vi "_Construct Lens Values.vi"(7 "Lens List":i32[](array[numeric])) -> (2 "# of Lens":i32, 3 "Table":string[][](table))   [LabVIEW 2012]
uses:
  Type/_Run Module.ctl
  Configuration/_Global Configuration.vi
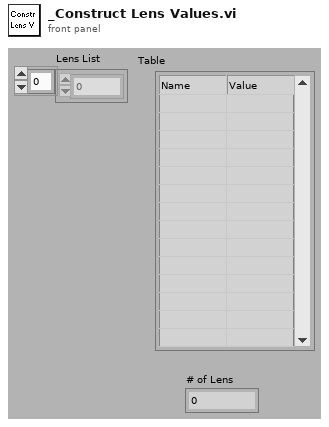
[diagram p1: front panel]
types:
  T1 = typedef "_Run Module.ctl" = u16
  T2 = typedef "_Lens Property.ctl" = cluster{"Scan Type":u8, "Scans":i32, "Time 1":dbl, "Time 2":dbl, "Value 1":dbl, "Value 2":dbl, "Step Size":dbl}
  T3 = typedef "_Mass Range Property.ctl" = cluster{"Start":dbl, "Stop":dbl, "Step Size":dbl, "Steps":i32, "Dwell":dbl, "Parameters":T4[], "Res":T5}
  T4 = typedef "_Mass Range Parameters.ctl" = cluster{"Name":string, "Ch#":u8, "StartV":dbl, "StopV":dbl, "StepV":dbl, "Index":u8}
  T5 = typedef "_RT Res Type.ctl" = u16
  T6 = typedef "_Run Mode.ctl" = enum16{"MRM (Q1/Q2)", "Q1 Scan", "Q1 SRM", "Q2 Scan", "Q2 SRM", "Product Scan", "Precursor Scan", "Neutral Loss", "Neutral Gain"}
  T7 = cluster{"Lenses":T2[], "Mass Ranges":T3[], "Acquire":bool, "MCA":bool, "Q1DC EN":bool, "Q1 POL":bool, "Q3 POL":bool, "Q1 RF  EN":bool, "Averaging":bool, "Log Scale":bool, "CPS":bool, "Unit":bool, "Data Path":path, "Run Mode":T6, "Fixed Mass (amu)":dbl, "Q3DC EN":bool, "Q3 RF  EN":bool, "Negative":bool}
  T8 = typedef "_RT Configuration 2.ctl" = cluster{"Name":string, "Ch#":u8, "Min":dbl, "Max":dbl, "Def+":dbl, "Def-":dbl, "Offset":dbl, "Slope":dbl, "Type":u8, "Description":string, "SettleT":dbl}
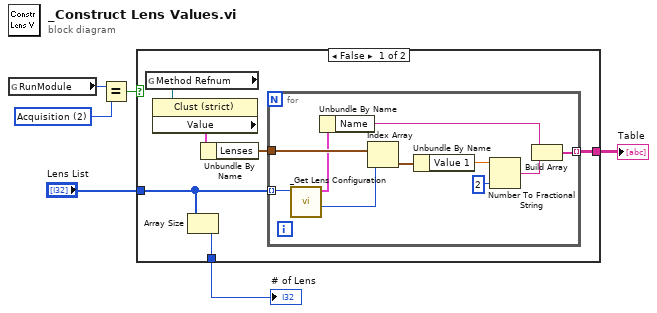
[diagram p0: block diagram]
diagram:
  w3 = T1 2 items=["Diagnostics", "Tune", "Acquisition"] ("y")
  n1 = global read "_Global Configuration.vi" "RunModule"() -> (w4:T1)
  n2 = Equal?(x=w4, y=w3) -> (x = y?=w2:bool)
  n3 = case shown="False" w2 {
    tunnel: [w9 _] -> w6
    tunnel: "Lens List" -> [w8 _]
    tunnel: [w7 _] -> w1
    frame False {
      n4 = global read "_Global Configuration.vi" "Method Refnum"() -> (w12:refnum<vi>)
      n5 = property class="Clust (strict)"(reference=w12) -> ("Value"=w11:T7)  [unwired: 1 in, 2 out]
      n6 = Array Size(array=w8) -> (size(s)=w7:i32)
      n7 = Unbundle By Name(w11) -> ("Lenses"=w10:T2[])
      n8 = for {
        tunnel: w8 -> [w22] mode=indexing
        tunnel: w10 -> [w21]
        tunnel: [w13] -> w9 mode=indexing
        n9 = call "_Get Lens Configuration.vi"("Channel #"=w22) -> ("Config Row#"=w20:i32, "Lens Configuration"=w18:T8)  [unwired: 1 in, 4 out]
        n10 = Unbundle By Name(w18) -> ("Name"=w15:string)
        n11 = Index Array(array=w21, index=w20) -> (element=w19:T2)
        n12 = Unbundle By Name(w19) -> ("Value 1"=w16:dbl)
        n13 = Number To Fractional String(number=w16, precision (6)=i16 2) -> (F-format string=w14:string)  [unwired: 2 out]
        n14 = Build Array(w15, w14) -> (w13:string[])
      }
    }
    frame True {
    }
  }
  "# of Lens" <- w1
  "Table" <- w6
